vi "InterpHoles.vi"(1 "min value":dbl format="%.2f", 2 "Interp Mode":i32=1, 3 "input array":dbl[](array[numeric]) format="%.2f") -> (0 "output array":dbl[](array[numeric]) format="%.2f")   [LabVIEW 2022 SP3]
uses:
  <vilib>/Analysis/NI_AALPro.lvlib
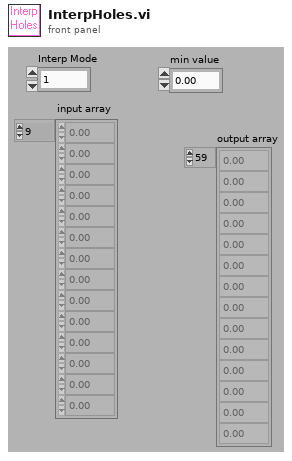
[diagram p1: front panel]
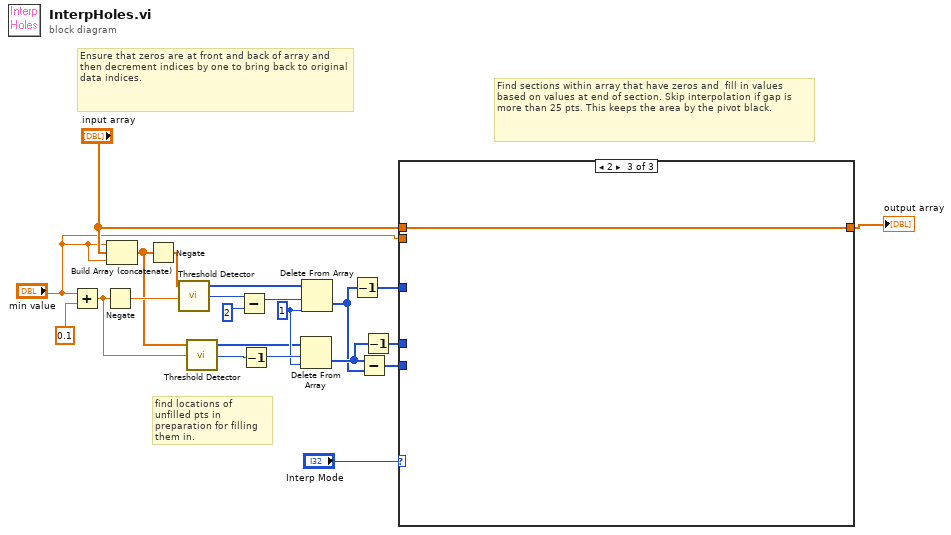
[diagram p0: block diagram]
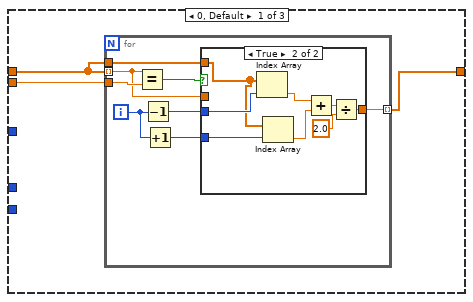
[diagram p2: hidden frame]
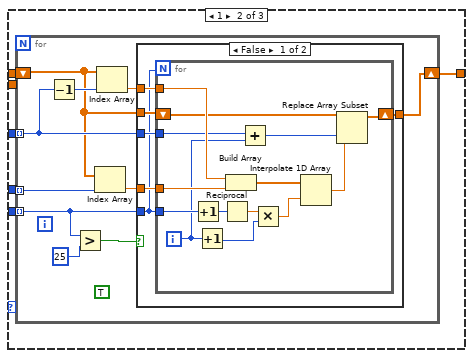
[diagram p4: hidden frame]
diagram:
  w13 = 1
  # "find locations of unfilled pts in preparation for filling them in."
  # "Ensure that zeros are at front and back of array and then decrement indices by one to bring back to original data indices."
  # "Find sections within array that have zeros and  fill in values based on values at end of section. Skip interpolation if gap is more than 25 pts. This keeps the area by the pivot black."
  n1 = Add(x="min value", y=0.1) -> (x+y=w21:dbl)
  n2 = Negate(x=w21) -> (-x=w22:dbl)
  n3 = Build Array (concatenate)("min value", "input array", "min value") -> (w12:dbl[])
  n4 = Negate(x=w12) -> (-x=w5:dbl[])
  n5 = call <vilib>:"Threshold Detector.vi"("threshold"=w22, "X"=w5) -> ("count"=w20:i32, "Indices"=w11:i32[])  [unwired: 1 in, 1 out]
  n6 = call <vilib>:"Threshold Detector.vi"("threshold"=w21, "X"=w12) -> ("count"=w17:i32, "Indices"=w9:i32[])  [unwired: 1 in, 1 out]
  n7 = Subtract(x=w20, y=2) -> (x-y=w18:i32)
  n8 = Decrement(x=w17) -> (x-1=w16:i32)
  n9 = Delete From Array(array=w9, length=w16, index=w13) -> (deleted portion=w15:i32[])  [unwired: 1 out]
  n10 = Delete From Array(array=w11, length=w18, index=w13) -> (deleted portion=w14:i32[])  [unwired: 1 out]
  n11 = Decrement(x=w14) -> (x-1=w8:i32[])
  n12 = Subtract(x=w15, y=w14) -> (x-y=w7:i32[])
  n13 = Decrement(x=w15) -> (x-1=w10:i32[])
  n14 = case shown="2" "Interp Mode" {
    tunnel: w10 -> [_ w47 _]
    tunnel: w8 -> [_ w46 _]
    tunnel: w7 -> [_ w45 _]
    tunnel: "input array" -> [w24 w44 w79]
    tunnel: [w23 w43 w79] -> w3
    tunnel: "min value" -> [w25 _ _]
    frame 0, Default {
      n15 = for {
        tunnel: w24 -> [w26] mode=indexing
        tunnel: w25 -> [w33]
        tunnel: w24 -> [w31]
        tunnel: [w27] -> w23 mode=indexing
        i -> [w29]
        n16 = Equal?(x=w26, y=w33) -> (x = y?=w32:bool)
        n17 = Decrement(x=w29) -> (x-1=w30:i32)
        n18 = Increment(x=w29) -> (x+1=w28:i32)
        n19 = case shown="True" w32 {
          tunnel: w31 -> [_ w39]
          tunnel: w30 -> [_ w42]
          tunnel: w28 -> [_ w41]
          tunnel: [w34 w35] -> w27
          tunnel: w26 -> [w34 _]
          frame False {
          }
          frame True {
            n20 = Index Array(array=w39, index=w42) -> (element=w40:dbl)
            n21 = Index Array(array=w39, index=w41) -> (element=w38:dbl)
            n22 = Add(x=w40, y=w38) -> (x+y=w37:dbl)
            n23 = Divide(x=w37, y=2.0) -> (x/y=w35:dbl)
          }
        }
      }
    }
    frame 1 {
      n24 = for {
        tunnel: w47 -> [w56] mode=indexing
        tunnel: w45 -> [w50] mode=indexing
        tunnel: w46 -> [w55] mode=indexing
        shift-right: [w51] -> w43
        shift-left: w44 -> [w52]
        (unwired) TRUE
        n25 = Decrement(x=w55) -> (x-1=w57:i32)
        n26 = Greater?(x=w50, y=25) -> (0:w48:bool)
        n27 = Index Array(array=w52, index=w56) -> (element=w53:dbl)
        n28 = Index Array(array=w52, index=w57) -> (element=w54:dbl)
        n29 = case shown="False" w48 {
          tunnel: w55 -> [w63 _]
          tunnel: w54 -> [w62 _]
          tunnel: w53 -> [w61 _]
          tunnel: w52 -> [w60 w78]
          tunnel: [w59 w78] -> w51
          tunnel: w50 -> [w58 _]
          frame False {
            n30 = for {
              N: w58 -> [_]
              tunnel: w63 -> [w67]
              tunnel: w58 -> [w77]
              tunnel: w62 -> [w75]
              tunnel: w61 -> [w74]
              shift-right: [w68] -> w59
              shift-left: w60 -> [w69]
              i -> [w64]
              n31 = Increment(x=w77) -> (x+1=w76:i32)
              n32 = Increment(x=w64) -> (x+1=w65:i32)
              n33 = Reciprocal(x=w76) -> (1/x=w72:dbl)
              n34 = Build Array(w75, w74) -> (w73:dbl[])
              n35 = Add(x=w67, y=w64) -> (x+y=w66:i32)
              n36 = Multiply(x=w72, y=w65) -> (x*y=w71:dbl)
              n37 = Interpolate 1D Array(1:w71, 2:w73) -> (0:w70:dbl)
              n38 = Replace Array Subset(array=w69, new element=w70, index=w66) -> (w68:dbl[])
            }
          }
          frame True {
          }
        }
      }
    }
    frame 2 {
    }
  }
  "output array" <- w3
